vi "Route To State.vi"(8 "error in":errorcluster, 9 "Outcome":string, 10 "Current State":string, 11 "Message Queue in":refnum<class "Delacor_lib_QMH_Message Queue.lvclass">) -> (0 "error out":errorcluster)   [LabVIEW 2021, in "Sequence Engine.lvlib"]
uses:
  Sequence Engine.lvlib
  <vilib>/Delacor/Delacor QMH/Libraries/Message Queue_class/Delacor_lib_QMH_Message Queue.lvclass
  <vilib>/Delacor/Delacor QMH/Libraries/Message Queue_class/Delacor_lib_QMH_Message Queue.lvclass/Delacor_lib_QMH_Message Queue.ctl
  <vilib>/Delacor/Delacor QMH/Libraries/Message Queue_class/Delacor_lib_QMH_Enqueue Message (Single).vi
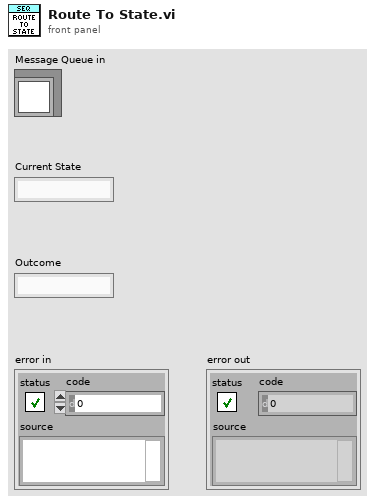
[diagram p1: front panel]
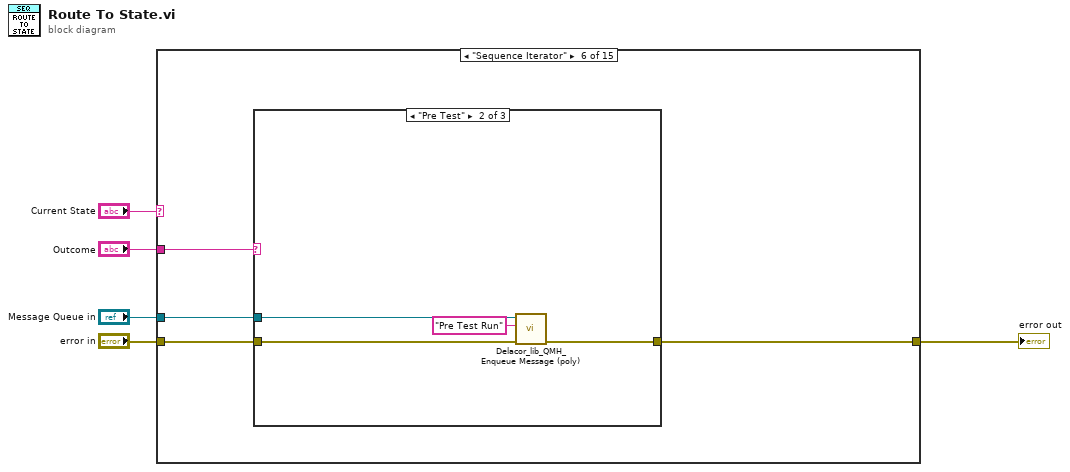
[diagram p0: block diagram]
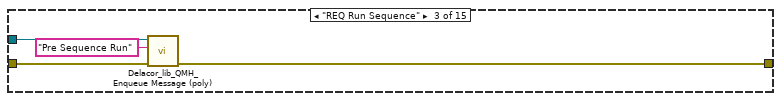
[diagram p4: hidden frame]
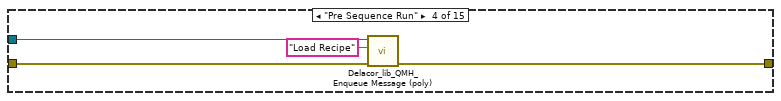
[diagram p5: hidden frame]
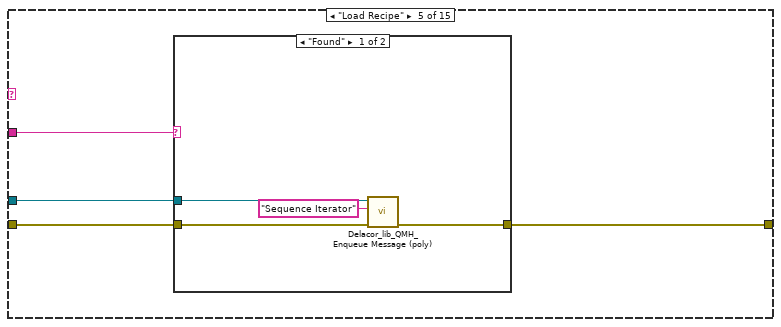
[diagram p6: hidden frame]
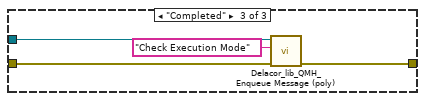
[diagram p9: hidden frame]
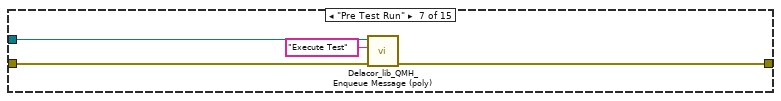
[diagram p10: hidden frame]
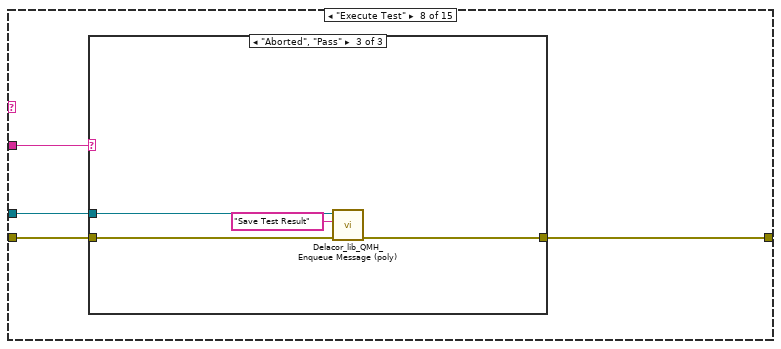
[diagram p11: hidden frame]
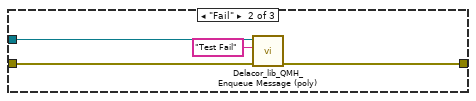
[diagram p13: hidden frame]
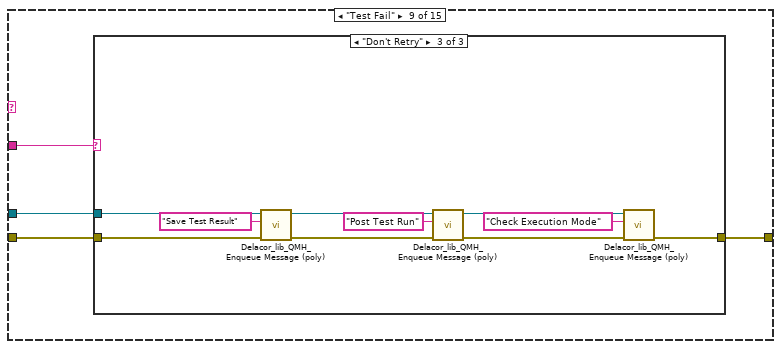
[diagram p14: hidden frame]
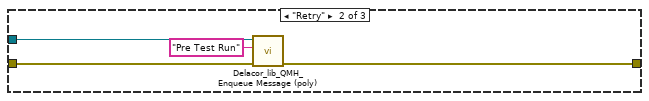
[diagram p16: hidden frame]
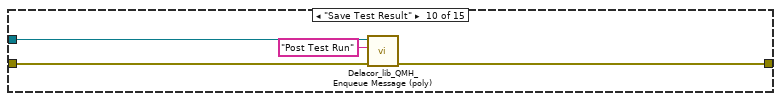
[diagram p17: hidden frame]
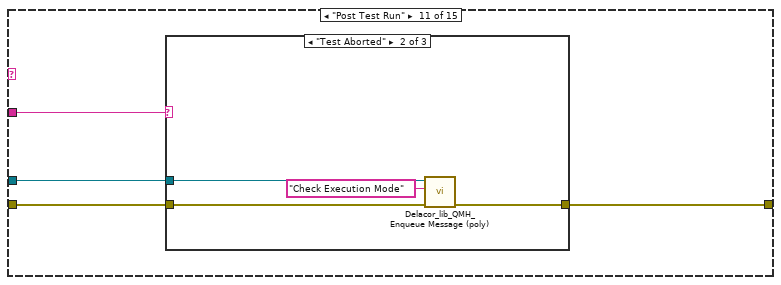
[diagram p18: hidden frame]
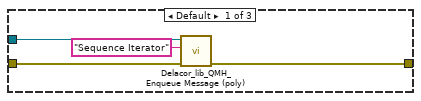
[diagram p19: hidden frame]
diagram:
  n1 = case shown="\"Sequence Iterator\"" "Current State" {
    tunnel: "Message Queue in" -> [_ _ w10 w13 w18 w27 w40 w45 w58 w76 w81 w94 w103 w107 w113]
    tunnel: "error in" -> [w6 w7 w9 w14 w19 w28 w41 w44 w57 w77 w80 w93 w102 w106 w109]
    tunnel: [w6 w7 w8 w12 w17 w26 w39 w43 w56 w75 w79 w92 w101 w105 w110] -> w2
    tunnel: "Outcome" -> [_ _ _ _ w16 w25 _ w42 w55 _ w78 w91 _ _ _]
    frame Default {
    }
    frame "Init Test Context" {
    }
    frame "REQ Run Sequence" {
      n2 = call-poly <vilib>:"Delacor_lib_QMH_Enqueue Message (poly).vi"("error in"=w9, "Message"="Pre Sequence Run", "Message Queue in"=w10) -> ("error out"=w8:errorcluster)  [unwired: 7 in, 1 out]
    }
    frame "Pre Sequence Run" {
      n3 = call-poly <vilib>:"Delacor_lib_QMH_Enqueue Message (poly).vi"("error in"=w14, "Message"="Load Recipe", "Message Queue in"=w13) -> ("error out"=w12:errorcluster)  [unwired: 7 in, 1 out]
    }
    frame "Load Recipe" {
      n4 = case shown="\"Found\"" w16 {
        tunnel: w19 -> [w22 w24]
        tunnel: w18 -> [w21 _]
        tunnel: [w20 w24] -> w17
        frame "Found" {
          n5 = call-poly <vilib>:"Delacor_lib_QMH_Enqueue Message (poly).vi"("error in"=w22, "Message"="Sequence Iterator", "Message Queue in"=w21) -> ("error out"=w20:errorcluster)  [unwired: 7 in, 1 out]
        }
        frame Default {
        }
      }
    }
    frame "Sequence Iterator" {
      n6 = case shown="\"Pre Test\"" w25 {
        tunnel: w28 -> [w29 w32 w36]
        tunnel: w27 -> [_ w31 w35]
        tunnel: [w29 w30 w34] -> w26
        frame Default {
        }
        frame "Pre Test" {
          n7 = call-poly <vilib>:"Delacor_lib_QMH_Enqueue Message (poly).vi"("error in"=w32, "Message"="Pre Test Run", "Message Queue in"=w31) -> ("error out"=w30:errorcluster)  [unwired: 7 in, 1 out]
        }
        frame "Completed" {
          n8 = call-poly <vilib>:"Delacor_lib_QMH_Enqueue Message (poly).vi"("error in"=w36, "Message"="Check Execution Mode", "Message Queue in"=w35) -> ("error out"=w34:errorcluster)  [unwired: 7 in, 1 out]
        }
      }
    }
    frame "Pre Test Run" {
      n9 = call-poly <vilib>:"Delacor_lib_QMH_Enqueue Message (poly).vi"("error in"=w41, "Message"="Execute Test", "Message Queue in"=w40) -> ("error out"=w39:errorcluster)  [unwired: 7 in, 1 out]
    }
    frame "Execute Test" {
      n10 = case shown="\"Aborted\", \"Pass\"" w42 {
        tunnel: w45 -> [_ w50 w54]
        tunnel: w44 -> [w46 w49 w53]
        tunnel: [w46 w48 w52] -> w43
        frame Default {
        }
        frame "Fail" {
          n11 = call-poly <vilib>:"Delacor_lib_QMH_Enqueue Message (poly).vi"("error in"=w49, "Message"="Test Fail", "Message Queue in"=w50) -> ("error out"=w48:errorcluster)  [unwired: 7 in, 1 out]
        }
        frame "Aborted", "Pass" {
          n12 = call-poly <vilib>:"Delacor_lib_QMH_Enqueue Message (poly).vi"("error in"=w53, "Message"="Save Test Result", "Message Queue in"=w54) -> ("error out"=w52:errorcluster)  [unwired: 7 in, 1 out]
        }
      }
    }
    frame "Test Fail" {
      n13 = case shown="\"Don't Retry\"" w55 {
        tunnel: w58 -> [_ w63 w73]
        tunnel: w57 -> [w59 w62 w72]
        tunnel: [w59 w61 w69] -> w56
        frame Default {
        }
        frame "Retry" {
          n14 = call-poly <vilib>:"Delacor_lib_QMH_Enqueue Message (poly).vi"("error in"=w62, "Message"="Pre Test Run", "Message Queue in"=w63) -> ("error out"=w61:errorcluster)  [unwired: 7 in, 1 out]
        }
        frame "Don't Retry" {
          n15 = call-poly <vilib>:"Delacor_lib_QMH_Enqueue Message (poly).vi"("error in"=w72, "Message"="Save Test Result", "Message Queue in"=w73) -> ("error out"=w65:errorcluster, "Message Queue out"=w66:refnum<class "Delacor_lib_QMH_Message Queue.lvclass">)  [unwired: 7 in]
          n16 = call-poly <vilib>:"Delacor_lib_QMH_Enqueue Message (poly).vi"("error in"=w65, "Message"="Post Test Run", "Message Queue in"=w66) -> ("error out"=w64:errorcluster, "Message Queue out"=w67:refnum<class "Delacor_lib_QMH_Message Queue.lvclass">)  [unwired: 7 in]
          n17 = call-poly <vilib>:"Delacor_lib_QMH_Enqueue Message (poly).vi"("error in"=w64, "Message"="Check Execution Mode", "Message Queue in"=w67) -> ("error out"=w69:errorcluster)  [unwired: 7 in, 1 out]
        }
      }
    }
    frame "Save Test Result" {
      n18 = call-poly <vilib>:"Delacor_lib_QMH_Enqueue Message (poly).vi"("error in"=w77, "Message"="Post Test Run", "Message Queue in"=w76) -> ("error out"=w75:errorcluster)  [unwired: 7 in, 1 out]
    }
    frame "Post Test Run" {
      n19 = case shown="\"Test Aborted\"" w78 {
        tunnel: w81 -> [w85 w89 _]
        tunnel: w80 -> [w84 w88 w90]
        tunnel: [w83 w87 w90] -> w79
        frame Default {
          n20 = call-poly <vilib>:"Delacor_lib_QMH_Enqueue Message (poly).vi"("error in"=w84, "Message"="Sequence Iterator", "Message Queue in"=w85) -> ("error out"=w83:errorcluster)  [unwired: 7 in, 1 out]
        }
        frame "Test Aborted" {
          n21 = call-poly <vilib>:"Delacor_lib_QMH_Enqueue Message (poly).vi"("error in"=w88, "Message"="Check Execution Mode", "Message Queue in"=w89) -> ("error out"=w87:errorcluster)  [unwired: 7 in, 1 out]
        }
        frame "Test Fail" {
        }
      }
    }
    frame "Check Execution Mode" {
      n22 = case shown="\"Production\"" w91 {
        tunnel: w94 -> [_ w99]
        tunnel: w93 -> [w95 w98]
        tunnel: [w95 w97] -> w92
        frame Default {
        }
        frame "Production" {
          n23 = call-poly <vilib>:"Delacor_lib_QMH_Enqueue Message (poly).vi"("error in"=w98, "Message"="Save Final Result", "Message Queue in"=w99) -> ("error out"=w97:errorcluster)  [unwired: 7 in, 1 out]
        }
      }
    }
    frame "Save Final Result" {
      n24 = call-poly <vilib>:"Delacor_lib_QMH_Enqueue Message (poly).vi"("error in"=w102, "Message"="Post Sequence Run", "Message Queue in"=w103) -> ("error out"=w101:errorcluster)  [unwired: 7 in, 1 out]
    }
    frame "Post Sequence Run" {
      n25 = call-poly <vilib>:"Delacor_lib_QMH_Enqueue Message (poly).vi"("error in"=w106, "Message"="Get UUT Serial Number", "Message Queue in"=w107) -> ("error out"=w105:errorcluster)  [unwired: 7 in, 1 out]
    }
    frame "Close All Modules" {
      n26 = call-poly <vilib>:"Delacor_lib_QMH_Enqueue Message (poly).vi"("Priority Message? (F)"=TRUE, "Message"="Exit", "Message Queue in"=w113) -> ("error out"=w112:errorcluster)  [unwired: 7 in, 1 out]
      n27 = Merge Errors(w112, w109) -> (w110:errorcluster)
    }
  }
  "error out" <- w2
